vi "BuildPlotColorsBands.vi"(5 "Labels":string[](array[string]), 6 "View Type":u16(ring) items=["As measured", "Normalize", "Separate", "Cplx Average", "Real Average", "Standard Deviation"], 7 "Colors":u32[](array[numeric]), 8 "error in (no error)":errorcluster, 9 "Bands":u16, 11 "WaveformGraph in":refnum<vi>) -> (3 "WaveformGraph out":refnum<vi>)   [LabVIEW 2022 SP3]
uses:
  Mic/Mic_Global.vi
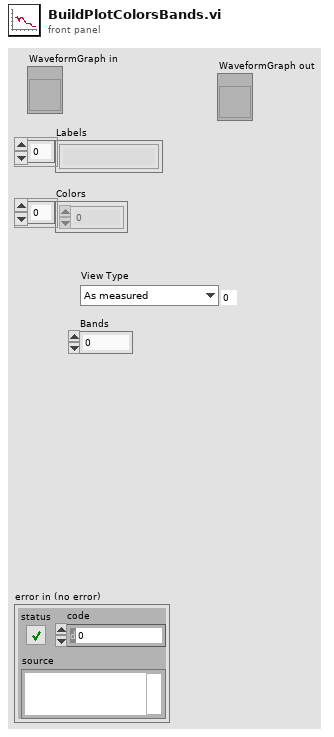
[diagram p1: front panel]
types:
  T1 = cluster{"Alerts":bool, "Log X Axis":bool, "dB scale":bool, "Averaging":bool, "Fade":dbl, "Centroids?":bool}
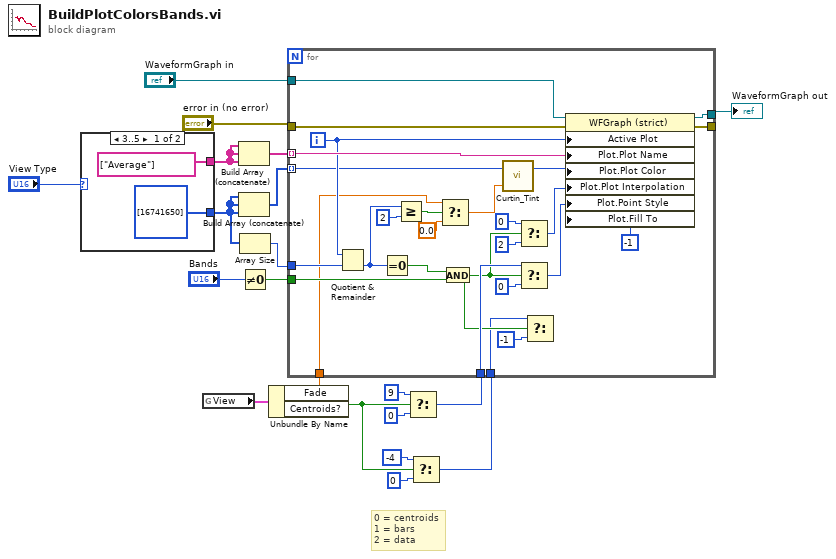
[diagram p0: block diagram]
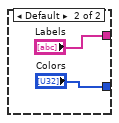
[diagram p2: hidden frame]
diagram:
  # "0 = centroids\n1 = bars\n2 = data"
  n1 = case shown="3..5" "View Type" {
    tunnel: [string[] ["Average"] ("Labels") "Labels"] -> w12
    tunnel: [u32[] [16741650] ("Colors") "Colors"] -> w11
    frame 3..5 {
    }
    frame Default {
    }
  }
  n2 = global read "Mic_Global.vi" "View"() -> (w10:T1)
  n3 = Build Array (concatenate)(w12, w12, w12) -> (w17:string[])
  n4 = Build Array (concatenate)(w11, w11, w11) -> (w14:u32[])
  n5 = Array Size(array=w11) -> (size(s)=w15:i32)
  n6 = Not Equal To 0?(x="Bands") -> (x != 0?=w20:bool)
  n7 = Unbundle By Name(w10) -> ("Fade"=w6:dbl, "Centroids?"=w3:bool)
  n8 = Select(t=9 ("y"), s=w3, f=0 ("y")) -> (s? t:f=w7:i32)
  n9 = Select(t=-4 ("y"), s=w3, f=0 ("y")) -> (s? t:f=w2:i32)
  n10 = for {
    tunnel: w14 -> [w31] mode=indexing
    tunnel: "WaveformGraph in" -> [w51]
    tunnel: w15 -> [w42]
    tunnel: "error in (no error)" -> [w47]
    tunnel: [w46] -> _
    tunnel: w17 -> [w45] mode=indexing
    tunnel: [w44] -> w18
    tunnel: w20 -> [w39]
    tunnel: w7 -> [w30]
    tunnel: w6 -> [w29]
    tunnel: w2 -> [w26]
    i -> [w43]
    n11 = Quotient & Remainder(x=w43, y=w42) -> (floor(x/y)=w38:i32)  [unwired: 1 out]
    n12 = Equal To 0?(x=w38) -> (x = 0?=w37:bool)
    n13 = Greater Or Equal?(x=w38, y=2) -> (x >= y?=w41:bool)
    n14 = Select(t=w29, s=w41, f=0.0 ("t")) -> (s? t:f=w50:dbl)
    n15 = And(x=w37, y=w39) -> (x .and. y?=w27:bool)
    n16 = call "Curtin_Tint.vi"("Tint Factor"=w50, "Plot.Plot Color"=w31) -> ("Plot.Plot Color 2"=w48:u32)  [unwired: 1 in]
    n17 = Select(t=0 ("y"), s=w27, f=2 ("y")) -> (s? t:f=w32:i32)
    n18 = Select(t=w30, s=w27, f=0 ("y")) -> (s? t:f=w35:i32)
    n19 = Select(t=w26, s=w27, f=-1 ("y")) -> ()  [unwired: 1 out]
    n20 = property on="Property Node" class="WFGraph (strict)"(reference=w51, error in=w47, "Active Plot"=w43, "Plot.Plot Name"=w45, "Plot.Plot Color"=w48, "Plot.Plot Interpolation"=w32, "Plot.Point Style"=w35, "Plot.Fill To"=i16 -1) -> (reference out=w44:refnum<vi>, error out=w46:errorcluster)
  }
  "WaveformGraph out" <- w18
